vi "Close Device Core.vi"(8 "error in (no error)":errorcluster, 11 "LS218 in":refnum<class "LS218.lvclass">) -> (0 "error out":errorcluster, 3 "LS218 out":refnum<class "LS218.lvclass">)   [LabVIEW 2013, in "LS218.lvlib" / "LS218.lvclass"]
doc: "Close device driver connection."
uses:
  LS218.lvclass
  CSPP_Core/Actors/CS++DeviceActor/CS++DeviceActor.lvclass
  LS218.lvclass/LS218.ctl
  <instrlib>/Lake Shore Cryotronics 218/Lake Shore Cryotronics 218.lvlib
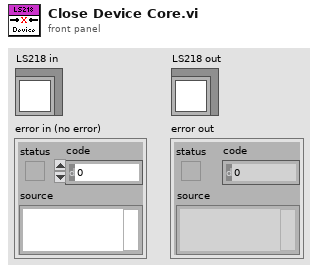
[diagram p1: front panel]
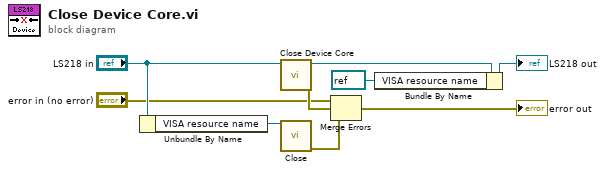
[diagram p0: block diagram]
diagram:
  n1 = Unbundle By Name("LS218 in") -> ("VISA resource name"=w7:refnum<visa-resource-name>)
  n2 = call-parent "Close Device Core.vi"("CS++DeviceActor in"="LS218 in") -> ("error out"=w9:errorcluster, "CS++DeviceActor out"=w3:refnum<class "LS218.lvclass">)  [unwired: 9 in]
  n3 = call <instrlib>:"Close.vi"("VISA resource name"=w7) -> ("error out"=w5:errorcluster)  [unwired: 14 in]
  n4 = Merge Errors("error in (no error)", w9, w5) -> (→"error out":errorcluster)
  n5 = Bundle By Name(cluster=w3, "VISA resource name"=refnum<visa-resource-name> refnum) -> (→"LS218 out":refnum<class "LS218.lvclass">)
